vi "Compare to masks new.vi"(5 "Temp Image":T1, 7 "Number of Particles1":i32=10, 8 "error in (no error)":errorcluster, 9 "Number of Particles":i32=1, 10 "Mask array":T1[](array[typedef]), 11 "Image Src":T1=refnum) -> (0 "Final error out":errorcluster={"status"=TRUE, "code"=-1074395995, "source"=""}, 3 "Marked Regions":bool[](array[boolean]))   [LabVIEW 2009]
doc: "From the marked regions, this VI outputs a one dimensional array of integers. Each element is a sector with a sick distance value in it. The 0th element represents the sector at 180 degrees, whlie the 29th element represents the sector at 0 degrees"
uses:
  <vilib>/vision/Image Controls.llb/IMAQ Image.ctl
  <vilib>/vision/NI_Vision_Development_Module.lvlib
panel:
  out "x < 0?":bool
  out "Erosion iteration":i32=3
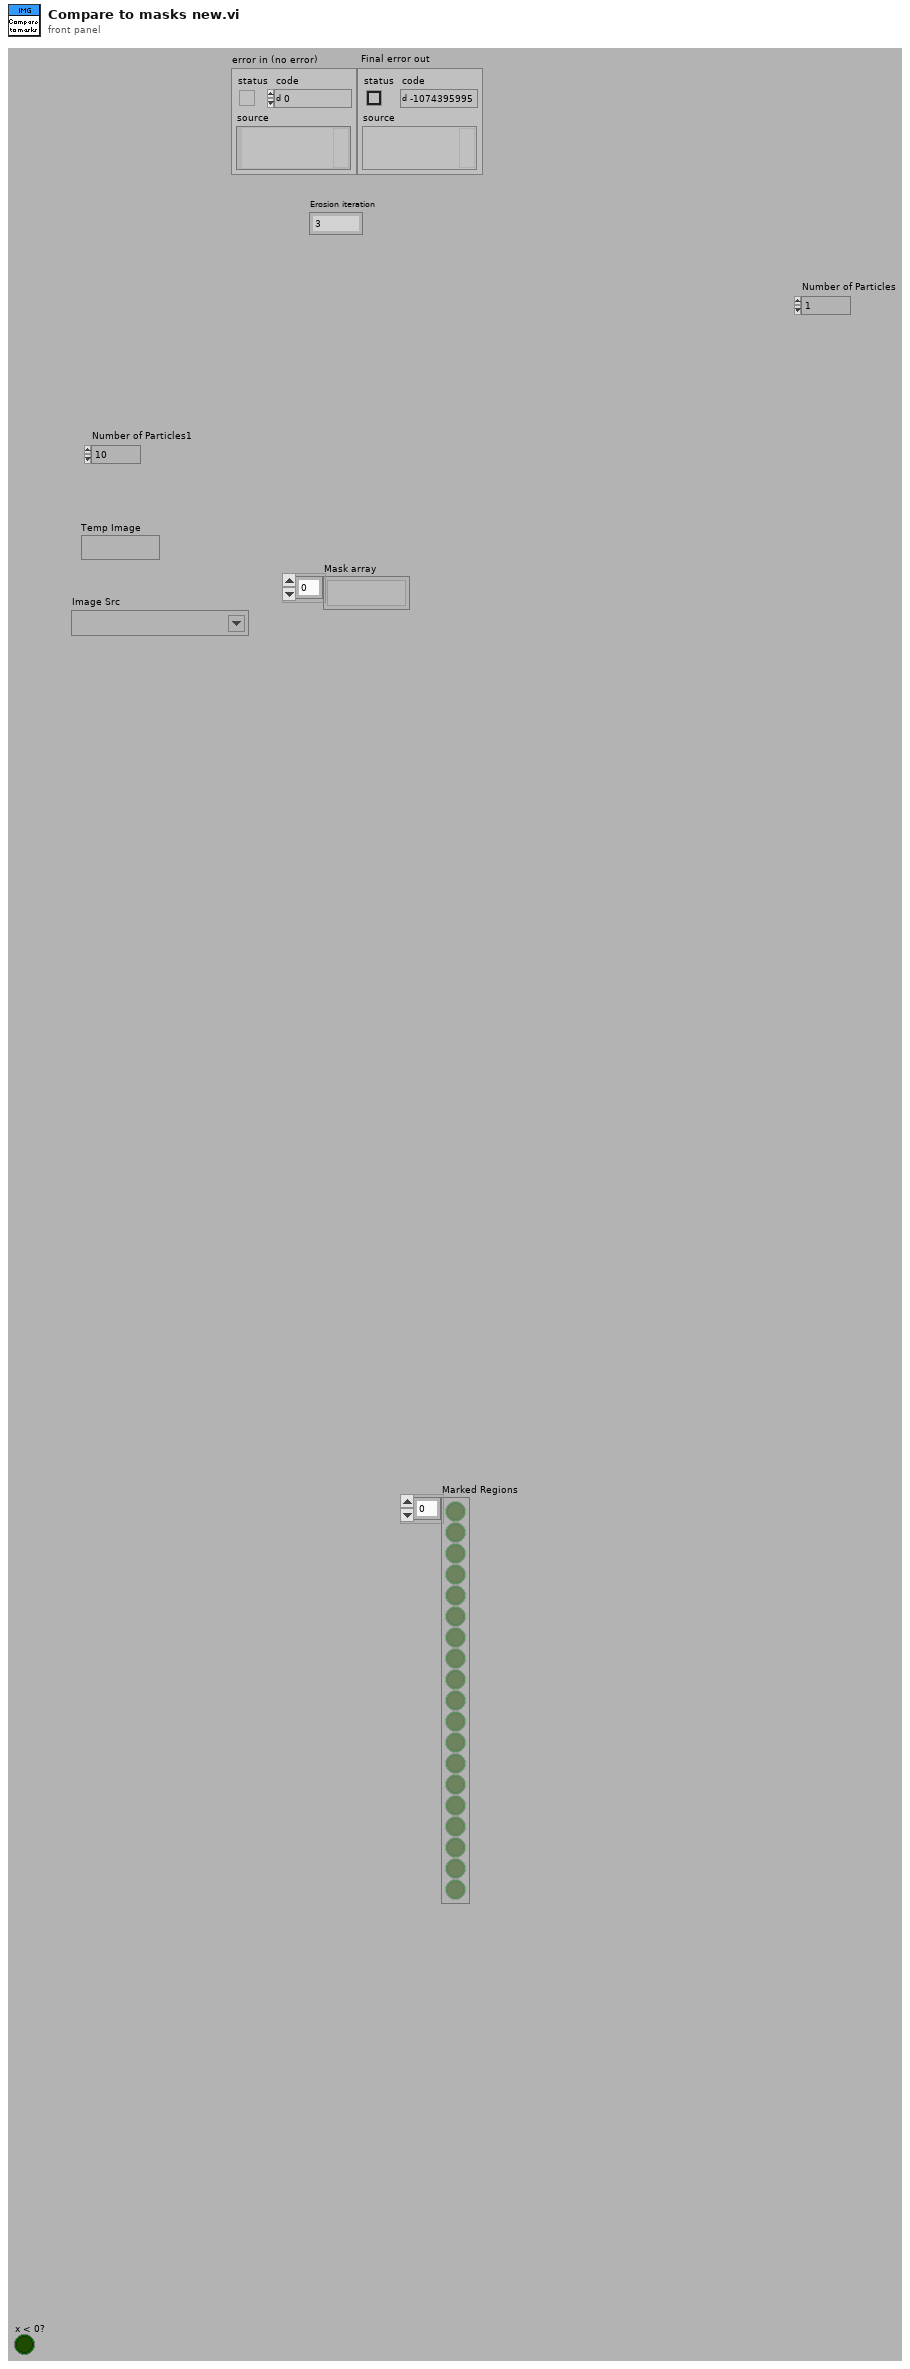
[diagram p1: front panel]
types:
  T1 = typedef "IMAQ Image.ctl" = refnum<image>
  T2 = enum32{"AutoM", "Close", "Dilate", "Erode", "Gradient", "Gradient out", "Gradient in", "Hit miss", "Open", "PClose", "POpen", "Thick", "Thin"}
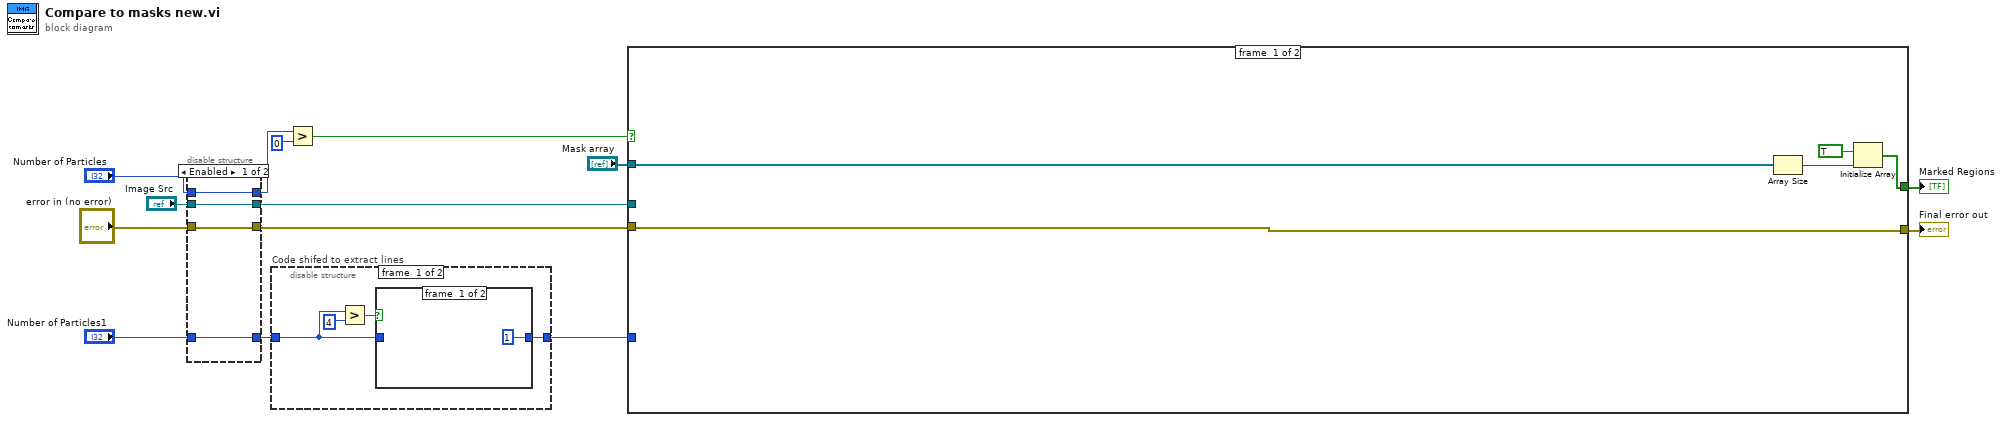
[diagram p0: block diagram]
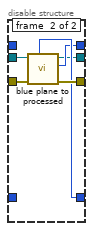
[diagram p2: hidden frame]
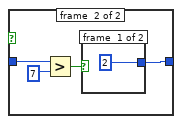
[diagram p3: hidden frame]
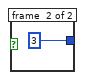
[diagram p4: hidden frame]
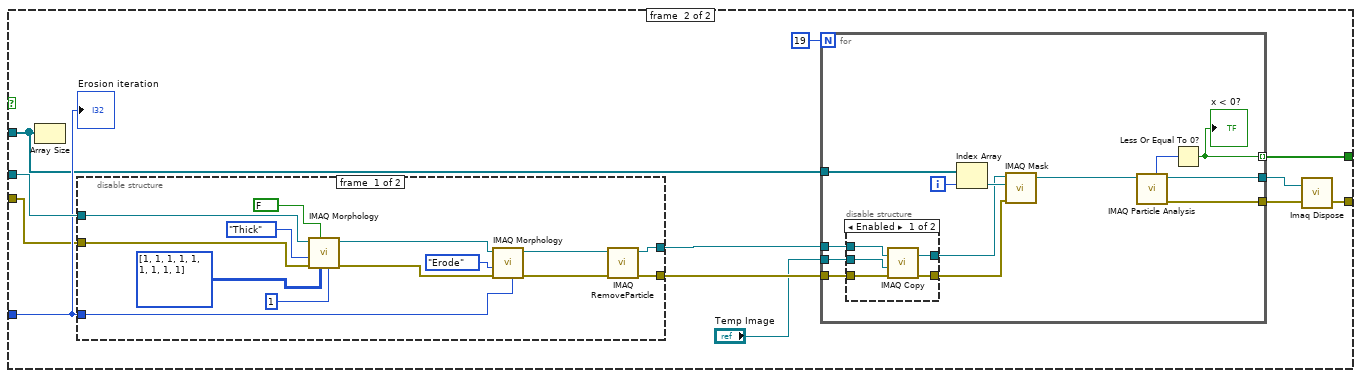
[diagram p6: hidden frame]
diagram:
  n1 = disable-structure shown="Enabled" {
    disable-tunnel: "error in (no error)" -> [w18 w24]
    disable-tunnel: [w18 w23] -> w8
    disable-tunnel: "Image Src" -> [w17 w22]
    disable-tunnel: [w17 w19] -> w1
    disable-tunnel: "Number of Particles" -> [w16 _]
    disable-tunnel: [w16 w20] -> w6
    disable-tunnel: [w15 w21] -> w5
    disable-tunnel: "Number of Particles1" -> [w15 _]
    frame #0 {
    }
    frame #1 {
      n2 = call "blue plane to processed.vi"("error in (no error)"=w24, "Image Src"=w22) -> ("error out"=w23:errorcluster, "Number of Particles"=w20:i32, "Image Dst Out"=w19:T1, "Number of Particles1"=w21:i32)  [unwired: 6 out]
    }
  }
  n3 = disable-structure "Code shifed to extract lines" shown="Enabled" {
    disable-tunnel: [w26 w36] -> w12
    disable-tunnel: w5 -> [w25 w36]
    frame #0 {
      n4 = Greater?(x=w25, y=4) -> (0:w27:bool)
      n5 = case shown="True" w27 {
        tunnel: [1 ("Number of iterations (1)") w31] -> w26
        tunnel: w25 -> [_ w33]
        frame #0 {
        }
        frame #1 {
          n6 = Greater?(x=w33, y=7) -> (0:w30:bool)
          n7 = case shown="True" w30 {
            tunnel: [2 ("Number of iterations (1)") 3 ("Number of iterations (1)")] -> w31
            frame #0 {
            }
            frame #1 {
            }
          }
        }
      }
    }
    frame #1 {
    }
  }
  n8 = Greater?(x=w6, y=0) -> (0:w14:bool)
  n9 = case shown="True" w14 {
    tunnel: w1 -> [_ w53]
    tunnel: w8 -> [w41 w50]
    tunnel: w12 -> [_ w52]
    tunnel: [w41 w48] -> w11
    tunnel: "Mask array" -> [w40 w51]
    tunnel: [w37 w47] -> w3
    frame #0 {
      n10 = Array Size(array=w40) -> (size(s)=w39:i32)
      n11 = Initialize Array(TRUE, w39) -> (w37:bool[])
    }
    frame #1 {
      n12 = Array Size(array=w51) -> ()  [unwired: 1 out]
      n13 = disable-structure shown="Enabled" {
        disable-tunnel: w53 -> [w64 w69]
        disable-tunnel: [w58 w69] -> w45
        disable-tunnel: w52 -> [w57 _]
        disable-tunnel: w50 -> [w55 w68]
        disable-tunnel: [w54 w68] -> w43
        frame #0 {
          n14 = call "IMAQ Morphology"("Number of iterations (1)"=1, "Structuring Element"=i32[][] [[1, 1, 1], [1, 1, 1], [1, 1, 1]], "Square/Hexa (Square)"=FALSE, "error in (no error)"=w55, "Operation"=T2."Thick", "Image Src"=w64) -> ("error out"=w62:errorcluster, "Image Dst Out"=w61:T1)  [unwired: 1 in, 3 out]
          n15 = call "IMAQ Morphology"("Number of iterations (1)"=w57, "error in (no error)"=w62, "Operation"=T2."Erode", "Image Src"=w61) -> ("error out"=w60:errorcluster, "Image Dst Out"=w59:T1)  [unwired: 3 in, 3 out]
          n16 = call "IMAQ RemoveParticle"("error in (no error)"=w60, "Image Src"=w59) -> ("error out"=w54:errorcluster, "Image Dst Out"=w58:T1)  [unwired: 5 in, 3 out]
        }
        frame #1 {
        }
      }
      n17 = for {
        N: 19 -> [_]
        tunnel: w45 -> [w80]
        tunnel: w51 -> [w79]
        tunnel: w43 -> [w78]
        tunnel: "Temp Image" -> [w77]
        tunnel: [w76] -> w49
        tunnel: [w72] -> w44
        tunnel: [w75] -> w47 mode=indexing
        i -> [w74]
        n18 = disable-structure shown="Enabled" {
          disable-tunnel: [w87 w88] -> w81
          disable-tunnel: w80 -> [w86 w89]
          disable-tunnel: w78 -> [w85 w88]
          disable-tunnel: w77 -> [w84 _]
          disable-tunnel: [w83 w89] -> w71
          frame #0 {
            n19 = call "IMAQ Copy"("error in (no error)"=w85, "Image Dst"=w84, "Image Src"=w86) -> ("error out"=w87:errorcluster, "Image Dst Out"=w83:T1)  [unwired: 3 out]
          }
          frame #1 {
          }
        }
        n20 = Index Array(array=w79, index=w74) -> (element=w73:T1)
        n21 = call "IMAQ Mask"("error in (no error)"=w81, "Image Mask"=w73, "Image Src"=w71) -> ("Image Dst Out"=w70:T1)  [unwired: 1 in, 2 out]
        n22 = call "IMAQ Particle Analysis"("Image"=w70) -> ("error out"=w76:errorcluster, "Image Out (duplicate)"=w72:T1, "Number of Particles"=w82:i32)  [unwired: 4 in, 4 out]
        n23 = Less Or Equal To 0?(x=w82) -> (x <= 0?=w75:bool)
        "x < 0?" <- w75
      }
      n24 = call "Imaq Dispose"("Image"=w44, "error in (no error)"=w49) -> ("error out"=w48:errorcluster)  [unwired: 4 in]
      "Erosion iteration" <- w52
    }
  }
  "Final error out" <- w11
  "Marked Regions" <- w3
